vi "Read Water Level.vi"(11 "更新水位消息输入":refnum<class "Update Water Level Msg.lvclass">) -> (2 "水位":dbl, 3 "更新水位消息输出":refnum<class "Update Water Level Msg.lvclass">)   [LabVIEW 2015, in "Water Level.lvlib" / "Update Water Level Msg.lvclass"]
doc: "读取水槽中的水位信息。"
uses:
  Update Water Level Msg.lvclass
  Update Water Level Msg.lvclass/Update Water Level Msg.ctl
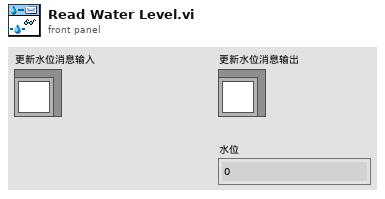
[diagram p1: front panel]
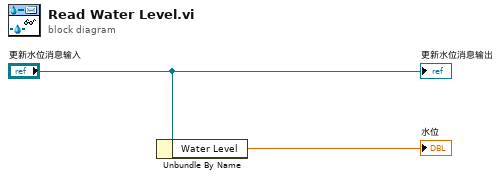
[diagram p0: block diagram]
diagram:
  n1 = Unbundle By Name("更新水位消息输入") -> ("Water Level"=→"水位":dbl)
  "更新水位消息输出" <- "更新水位消息输入"
